vi "Add Calculate Channel_Conditional_Conditional.vi"(7 "SysDef Ref":T1, 8 "error in (error out)":errorcluster, 9 "Conditional Settings":T2, 11 "Calculated Channels Ref":refnum<k24>) -> (0 "error out":errorcluster, 3 "Calculated Channels Ref Out":refnum<k24>)   [LabVIEW 2019, in "Simple SysDef API.lvlib"]
uses:
  <userlib>/SimpleSysDef/Simple SysDef API.lvlib
  NationalInstruments.VeriStand.SystemDefinitionAPI
  <userlib>/SimpleSysDef/_SubVIs/Add Calculate Channel_Conditional_Settings.ctl
  <userlib>/SimpleSysDef/_SubVIs/System Definition Reference.ctl
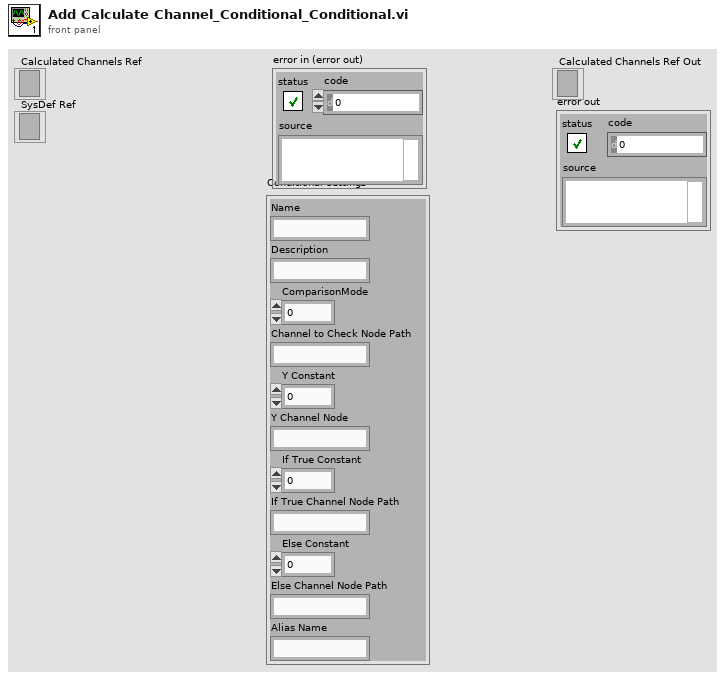
[diagram p1: front panel]
types:
  T1 = typedef "Simple SysDef API.lvlib/System Definition Reference.ctl" = refnum<k24>
  T2 = typedef "Simple SysDef API.lvlib/Add Calculate Channel_Conditional_Settings.ctl" = cluster{"Name":string, "Description":string, "ComparisonMode":u16, "Channel to Check Node Path":string, "Y Constant":dbl, "Y Channel Node":string, "If True Constant":dbl, "If True Channel Node Path":string, "Else Constant ":dbl, "Else Channel Node Path":string, "Alias Name":string}
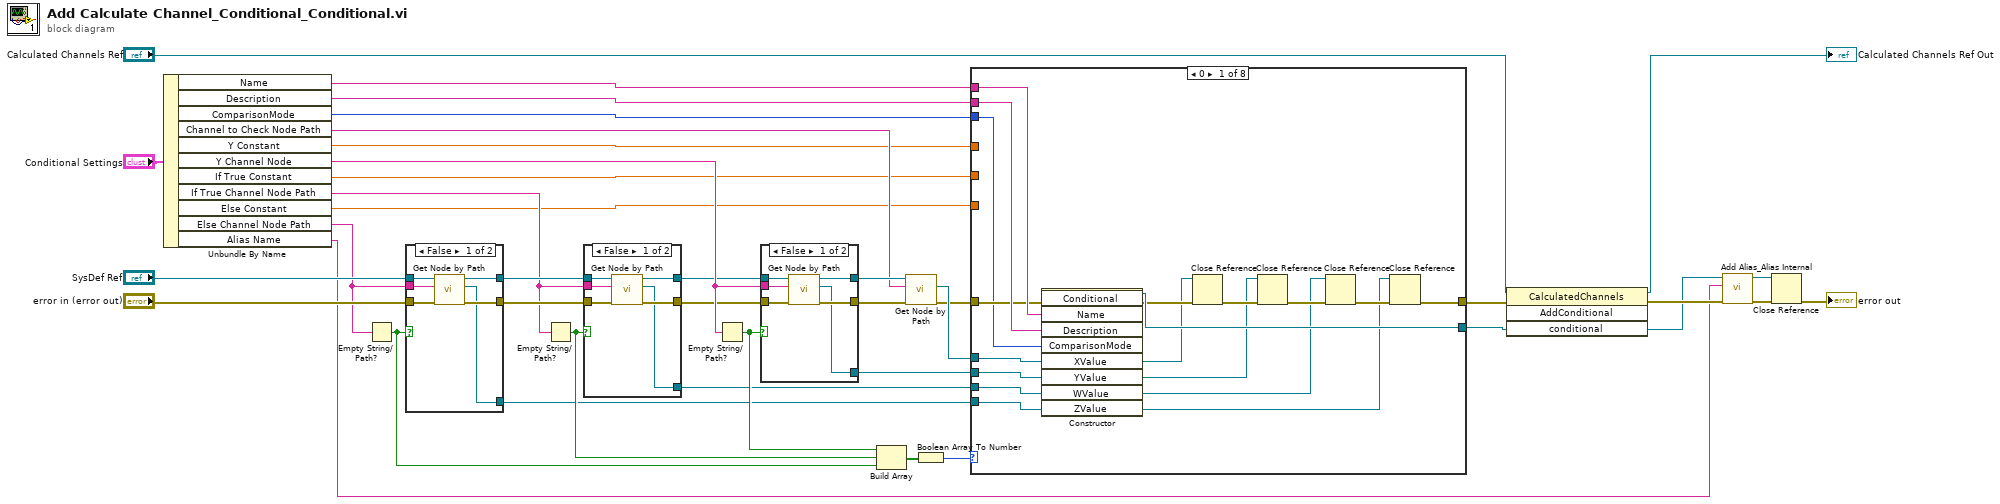
[diagram p0: block diagram]
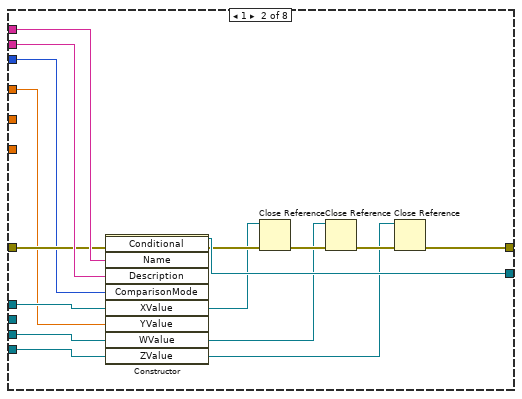
[diagram p4: hidden frame]
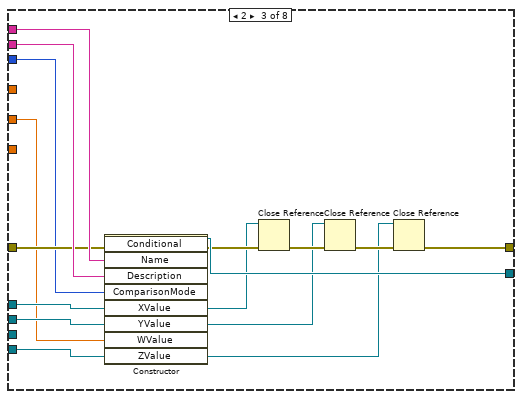
[diagram p5: hidden frame]
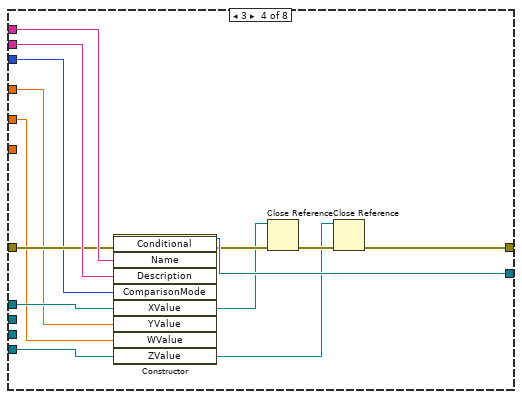
[diagram p6: hidden frame]
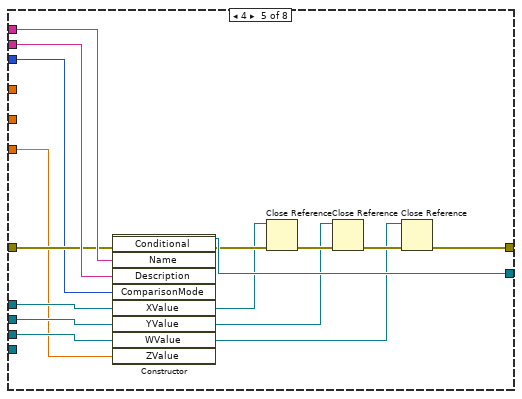
[diagram p7: hidden frame]
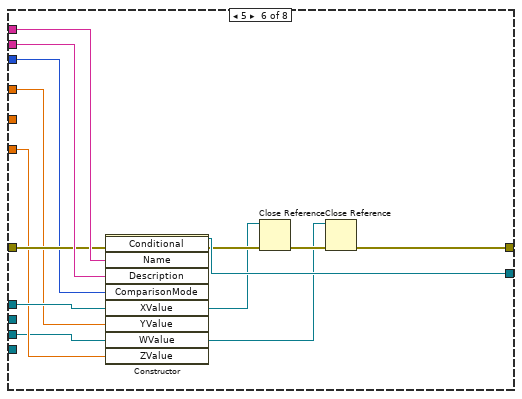
[diagram p8: hidden frame]
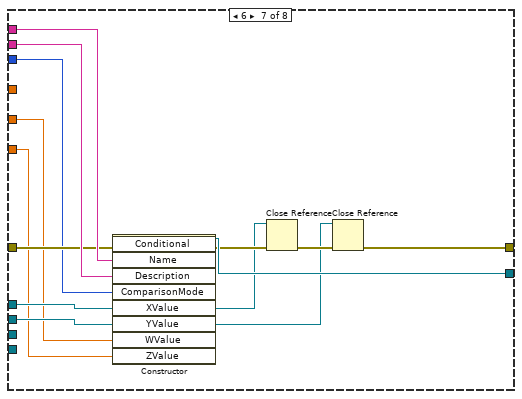
[diagram p9: hidden frame]
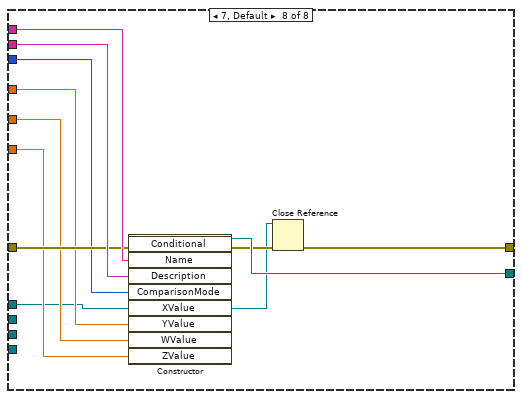
[diagram p10: hidden frame]
diagram:
  n1 = Unbundle By Name("Conditional Settings") -> ("Name"=w34:string, "Description"=w33:string, "ComparisonMode"=w7:u16, "Channel to Check Node Path"=w26:string, "Y Constant"=w21:dbl, "Y Channel Node"=w31:string, "If True Constant"=w9:dbl, "If True Channel Node Path"=w10:string, "Else Constant"=w8:dbl, "Else Channel Node Path"=w11:string, "Alias Name"=w1:string)
  n2 = Empty String/Path?(string/path=w11) -> (empty?=w14:bool)
  n3 = case shown="False" w14 {
    tunnel: "error in (error out)" -> [w44 w46]
    tunnel: [w43 w46] -> w19
    tunnel: "SysDef Ref" -> [w42 w45]
    tunnel: [w41 w45] -> w20
    tunnel: [w40 _] -> w6
    tunnel: w11 -> [w39 _]
    frame False {
      n4 = call <userlib>:"Get Node by Path.vi"("error in (no error)"=w44, "System Definition Node Path"=w39, "SysDef Ref"=w42) -> ("error out"=w43:errorcluster, "Node Ref"=w40:refnum<k24>, "SysDef Ref Out"=w41:T1)  [unwired: 6 in]
    }
    frame True {
    }
  }
  n5 = Empty String/Path?(string/path=w10) -> (empty?=w15:bool)
  n6 = case shown="False" w15 {
    tunnel: w19 -> [w52 w54]
    tunnel: [w51 w54] -> w18
    tunnel: w20 -> [w50 w53]
    tunnel: [w49 w53] -> w17
    tunnel: [w48 _] -> w16
    tunnel: w10 -> [w47 _]
    frame False {
      n7 = call <userlib>:"Get Node by Path.vi"("error in (no error)"=w52, "System Definition Node Path"=w47, "SysDef Ref"=w50) -> ("error out"=w51:errorcluster, "Node Ref"=w48:refnum<k24>, "SysDef Ref Out"=w49:T1)  [unwired: 6 in]
    }
    frame True {
    }
  }
  n8 = Empty String/Path?(string/path=w31) -> (empty?=w25:bool)
  n9 = case shown="False" w25 {
    tunnel: w18 -> [w60 w62]
    tunnel: [w59 w62] -> w29
    tunnel: w17 -> [w58 w61]
    tunnel: [w57 w61] -> w30
    tunnel: [w56 _] -> w32
    tunnel: w31 -> [w55 _]
    frame False {
      n10 = call <userlib>:"Get Node by Path.vi"("error in (no error)"=w60, "System Definition Node Path"=w55, "SysDef Ref"=w58) -> ("error out"=w59:errorcluster, "Node Ref"=w56:refnum<k24>, "SysDef Ref Out"=w57:T1)  [unwired: 6 in]
    }
    frame True {
    }
  }
  n11 = Build Array(w25, w15, w14) -> (w24:bool[])
  n12 = call <userlib>:"Get Node by Path.vi"("error in (no error)"=w29, "System Definition Node Path"=w26, "SysDef Ref"=w30) -> ("error out"=w27:errorcluster, "Node Ref"=w28:refnum<k24>)  [unwired: 6 in, 1 out]
  n13 = Boolean Array To Number(Boolean array=w24) -> (number=w23:u32)
  n14 = case shown="0" w23 {
    tunnel: [w66 w81 w93 w107 w116 w131 w141 w153] -> w22
    tunnel: [w76 w89 w102 w114 w127 w139 w151 w155] -> w3
    tunnel: w34 -> [w75 w88 w101 w113 w126 w138 w150 w162]
    tunnel: w33 -> [w74 w87 w100 w112 w125 w137 w149 w161]
    tunnel: w32 -> [w70 _ w96 _ w121 _ w145 _]
    tunnel: w28 -> [w69 w83 w95 w108 w120 w133 w144 w152]
    tunnel: w27 -> [w73 w86 w99 w111 w124 w136 w148 w160]
    tunnel: w21 -> [_ w78 _ w106 _ w130 _ w158]
    tunnel: w16 -> [w65 w79 _ _ w118 w129 _ _]
    tunnel: w6 -> [w64 w80 w92 w105 _ _ _ _]
    tunnel: w9 -> [_ _ w91 w104 _ _ w142 w157]
    tunnel: w8 -> [_ _ _ _ w117 w132 w143 w156]
    tunnel: w7 -> [w63 w77 w90 w103 w115 w128 w140 w159]
    frame 0 {
      n15 = constructor class="Conditional"(error in=w73, "Name"=w75, "Description"=w74, "ComparisonMode"=w63, "XValue"=w69, "YValue"=w70, "WValue"=w65, "ZValue"=w64) -> (reference out=w76:refnum<k24>, error out=w71:errorcluster)  [unwired: 2 in, 8 out]
      n16 = Close Reference(reference=w69, error in (no error)=w71) -> (error out=w72:errorcluster)
      n17 = Close Reference(reference=w70, error in (no error)=w72) -> (error out=w67:errorcluster)
      n18 = Close Reference(reference=w65, error in (no error)=w67) -> (error out=w68:errorcluster)
      n19 = Close Reference(reference=w64, error in (no error)=w68) -> (error out=w66:errorcluster)
    }
    frame 1 {
      n20 = constructor class="Conditional"(error in=w86, "Name"=w88, "Description"=w87, "ComparisonMode"=w77, "XValue"=w83, "YValue"=w78, "WValue"=w79, "ZValue"=w80) -> (reference out=w89:refnum<k24>, error out=w84:errorcluster)  [unwired: 2 in, 8 out]
      n21 = Close Reference(reference=w83, error in (no error)=w84) -> (error out=w85:errorcluster)
      n22 = Close Reference(reference=w79, error in (no error)=w85) -> (error out=w82:errorcluster)
      n23 = Close Reference(reference=w80, error in (no error)=w82) -> (error out=w81:errorcluster)
    }
    frame 2 {
      n24 = constructor class="Conditional"(error in=w99, "Name"=w101, "Description"=w100, "ComparisonMode"=w90, "XValue"=w95, "YValue"=w96, "WValue"=w91, "ZValue"=w92) -> (reference out=w102:refnum<k24>, error out=w97:errorcluster)  [unwired: 2 in, 8 out]
      n25 = Close Reference(reference=w95, error in (no error)=w97) -> (error out=w98:errorcluster)
      n26 = Close Reference(reference=w96, error in (no error)=w98) -> (error out=w94:errorcluster)
      n27 = Close Reference(reference=w92, error in (no error)=w94) -> (error out=w93:errorcluster)
    }
    frame 3 {
      n28 = constructor class="Conditional"(error in=w111, "Name"=w113, "Description"=w112, "ComparisonMode"=w103, "XValue"=w108, "YValue"=w106, "WValue"=w104, "ZValue"=w105) -> (reference out=w114:refnum<k24>, error out=w109:errorcluster)  [unwired: 2 in, 8 out]
      n29 = Close Reference(reference=w108, error in (no error)=w109) -> (error out=w110:errorcluster)
      n30 = Close Reference(reference=w105, error in (no error)=w110) -> (error out=w107:errorcluster)
    }
    frame 4 {
      n31 = constructor class="Conditional"(error in=w124, "Name"=w126, "Description"=w125, "ComparisonMode"=w115, "XValue"=w120, "YValue"=w121, "WValue"=w118, "ZValue"=w117) -> (reference out=w127:refnum<k24>, error out=w122:errorcluster)  [unwired: 2 in, 8 out]
      n32 = Close Reference(reference=w120, error in (no error)=w122) -> (error out=w123:errorcluster)
      n33 = Close Reference(reference=w121, error in (no error)=w123) -> (error out=w119:errorcluster)
      n34 = Close Reference(reference=w118, error in (no error)=w119) -> (error out=w116:errorcluster)
    }
    frame 5 {
      n35 = constructor class="Conditional"(error in=w136, "Name"=w138, "Description"=w137, "ComparisonMode"=w128, "XValue"=w133, "YValue"=w130, "WValue"=w129, "ZValue"=w132) -> (reference out=w139:refnum<k24>, error out=w134:errorcluster)  [unwired: 2 in, 8 out]
      n36 = Close Reference(reference=w133, error in (no error)=w134) -> (error out=w135:errorcluster)
      n37 = Close Reference(reference=w129, error in (no error)=w135) -> (error out=w131:errorcluster)
    }
    frame 6 {
      n38 = constructor class="Conditional"(error in=w148, "Name"=w150, "Description"=w149, "ComparisonMode"=w140, "XValue"=w144, "YValue"=w145, "WValue"=w142, "ZValue"=w143) -> (reference out=w151:refnum<k24>, error out=w146:errorcluster)  [unwired: 2 in, 8 out]
      n39 = Close Reference(reference=w144, error in (no error)=w146) -> (error out=w147:errorcluster)
      n40 = Close Reference(reference=w145, error in (no error)=w147) -> (error out=w141:errorcluster)
    }
    frame 7, Default {
      n41 = constructor class="Conditional"(error in=w160, "Name"=w162, "Description"=w161, "ComparisonMode"=w159, "XValue"=w152, "YValue"=w158, "WValue"=w157, "ZValue"=w156) -> (reference out=w155:refnum<k24>, error out=w154:errorcluster)  [unwired: 2 in, 8 out]
      n42 = Close Reference(reference=w152, error in (no error)=w154) -> (error out=w153:errorcluster)
    }
  }
  n43 = invoke class="CalculatedChannels" method="AddConditional"(reference="Calculated Channels Ref", error in=w22, "conditional"=w3) -> (reference out=→"Calculated Channels Ref Out":refnum<k24>, error out=w5:errorcluster)  [unwired: 1 in, 2 out]
  n44 = call <userlib>:"Add Alias_Alias Internal.vi"("error in (no error)"=w5, "Name"=w1, "Base Node"=w3) -> ("error out"=w4:errorcluster, "Base Node out"=w2:refnum<k24>)  [unwired: 7 in]
  n45 = Close Reference(reference=w2, error in (no error)=w4) -> (error out=→"error out":errorcluster)
